vi "GenerateLogfilepath.vi"(1 "Instrument":string="Control") -> (0 "Logfile Path":path)   [LabVIEW 2018]
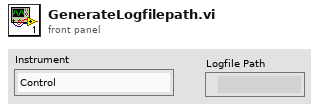
[diagram p1: front panel]
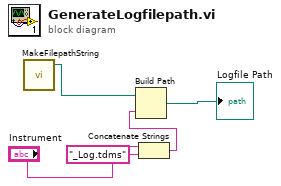
[diagram p0: block diagram]
diagram:
  n1 = call "MakeFilepathString.vi"() -> ("Date Folder"=w2:path)  [unwired: 5 in, 2 out]
  n2 = Concatenate Strings("Instrument", "_Log.tdms" ("string")) -> (w3:string)
  n3 = Build Path(base path=w2, name or relative path=w3) -> (appended path=→"Logfile Path":path)
